vi "Heartbeat.vi"() -> ()   [LabVIEW 2018]
uses:
  Libraries/AWS_IoT_Coms/AWS_IoT_Coms.lvlib
panel:
  out "ms":u32
  out "x >= y?":bool
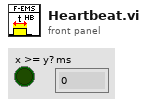
[diagram p1: front panel]
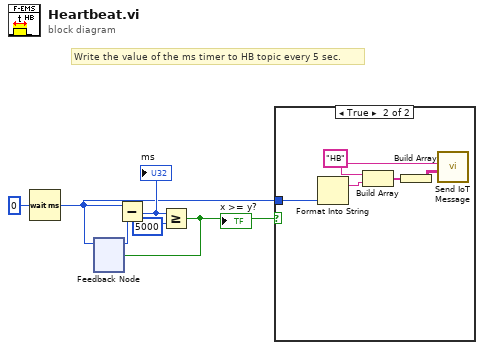
[diagram p0: block diagram]
diagram:
  # "Write the value of the ms timer to HB topic every 5 sec."
  n1 = Wait (ms)(milliseconds to wait=u32 0) -> (millisecond timer value=w1:u32)
  n2 = feedback #1() -> (w3:u32)  [unwired: 1 in]
  n3 = Subtract(x=w1, y=w3) -> (x-y=w6:u32)
  "ms" <- w6
  n4 = Greater Or Equal?(x=w6, y=u32 5000) -> (x >= y?=w4:bool)
  "x >= y?" <- w4
  n5 = feedback-in #1(w1, w4) -> ()
  n6 = case shown="True" w4 {
    tunnel: w1 -> [_ w11]
    frame False {
    }
    frame True {
      w7 = "HB" ("Topic")
      n7 = Format Into String(w11) -> (resulting string=w10:string)  [unwired: 3 in, 1 out]
      n8 = Build Array(w7, w10) -> (w9:string[])
      n9 = Build Array(w9) -> (w8:string[][])
      n10 = call "Send IoT Message.vi"("Name Value Pairs"=w8, "Topic"=w7) -> ()  [unwired: 9 in, 1 out]
    }
  }
